vi "parse_XML_string.vi"(7 "ID attribute":string="ID", 8 "error in (no error)":errorcluster, 10 "XML string":string, 11 "Element in":refnum<class "XMLElement.lvclass">) -> (0 "error out":errorcluster, 3 "Element out":refnum<class "XMLElement.lvclass">, 4 "header empty or invalid XML?":bool)   [LabVIEW 2010, in "XMLElement.lvclass"]
uses:
  XMLElement.lvclass
  XMLElement.lvclass/XMLElement.ctl
  Program Files (x86)/National Instruments/LabVIEW 2010/resource/objmgr/DOMUserDefRef.rc
  <vilib>/xml/NI_XML.lvlib
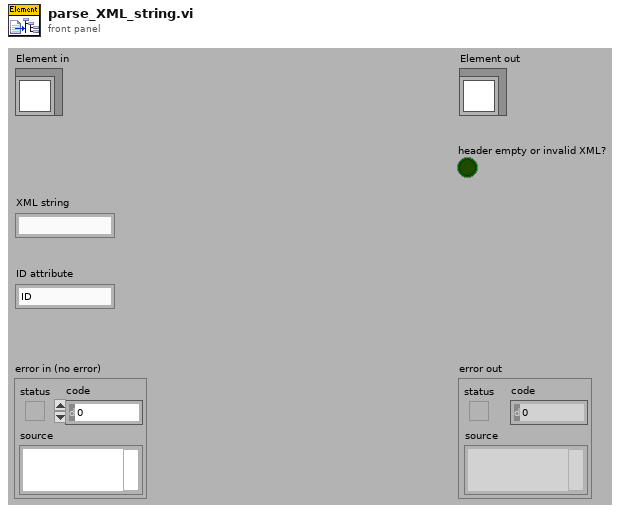
[diagram p1: front panel]
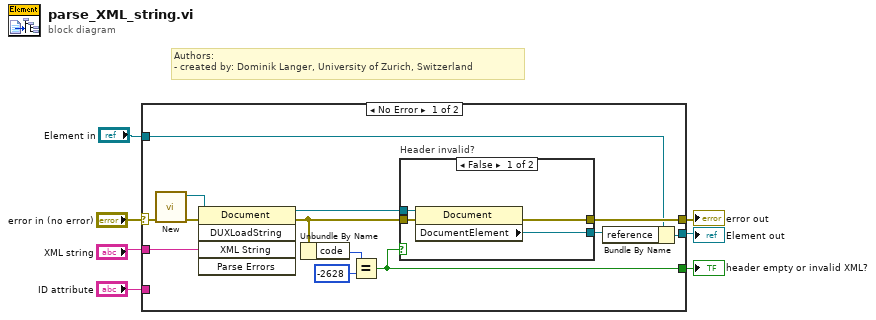
[diagram p0: block diagram]
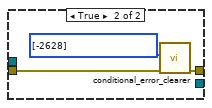
[diagram p2: hidden frame]
diagram:
  # "Authors: \n- created by: Dominik Langer, University of Zurich, Switzerland"
  n1 = case shown="No Error" "error in (no error)" {
    selector: "error in (no error)" -> [w16 w29]
    tunnel: [w13 w29] -> w7
    tunnel: [w8 w28] -> w6
    tunnel: "Element in" -> [w10 w28]
    tunnel: "XML string" -> [w18 _]
    tunnel: "ID attribute" -> [_ _]
    tunnel: [w11 _] -> w1
    frame No Error {
      n2 = call <vilib>:"New.vi"("error in (no error)"=w16) -> ("error out"=w20:errorcluster, "DOM document out"=w19:refnum<k20>)  [unwired: 7 in]
      n3 = invoke class="Document" method="DUXLoadString"(reference=w19, error in=w20, "XML String"=w18) -> (reference out=w17:refnum<k20>, error out=w12:errorcluster)  [unwired: 2 in, 3 out]
      n4 = Unbundle By Name(w12) -> ("code"=w14:i32)
      n5 = Equal?(x=w14, y=-2628) -> (x = y?=w11:bool)
      n6 = case "Header invalid?" shown="False" w11 {
        tunnel: w17 -> [w24 _]
        tunnel: [w23 w25] -> w13
        tunnel: w12 -> [w22 w26]
        tunnel: [w21 _] -> w9
        frame False {
          n7 = property class="Document"(reference=w24, error in=w22) -> (error out=w23:errorcluster, "DocumentElement"=w21:refnum<k20>)  [unwired: 1 out]
        }
        frame True {
          n8 = call "conditional_error_clearer.vi"("error in (no error)"=w26, "array of clearable error codes"=i32[] [-2628]) -> ("error out"=w25:errorcluster)  [unwired: 9 in]
        }
      }
      n9 = Bundle By Name(cluster=w10, "reference"=w9) -> (w8:refnum<class "XMLElement.lvclass">)
    }
    frame Error {
    }
  }
  "error out" <- w7
  "Element out" <- w6
  "header empty or invalid XML?" <- w1
